vi "test_Bitfile Reload_Speciality IO Data Type Change.vi"(8 "error in (no error)":errorcluster, 11 "TestCase in":refnum<class "FPGA Addon Bitfile Reload Unit Tests.lvclass">) -> (0 "error out":errorcluster, 3 "TestCase out":refnum<class "FPGA Addon Bitfile Reload Unit Tests.lvclass">)   [LabVIEW 2020, in "FPGA Addon Bitfile Reload Unit Tests.lvclass"]
uses:
  FPGA Addon Bitfile Reload Unit Tests.lvclass
  APIs/Scripting API/TypeDefs/Output Scalar Data.ctl
  Addon/Addon Shared/Types/FPGA Addon Data Type.ctl
  APIs/Scripting API/Public/Bitfile Resources/Import Bitfile Scalars (Instances)/Import Scalars - all.vi
  <vilib>/addons/_JKI Toolkits/VI Tester/TestCase.llb/TestCase.lvclass
  APIs/Scripting API/Scripting API.lvlib
  FPGA Addon Test Class/FPGA Addon Test Class.lvclass
  Addon/Addon System Explorer/FPGA Addon System Explorer.lvlib
  Addon/Addon Shared/FPGA Addon Shared.lvlib
  C:/Program Files (x86)/National Instruments/LabVIEW 2020/vi.lib/addons/_JKI Toolkits/VI Tester/TestCase.llb/TestCase.lvclass
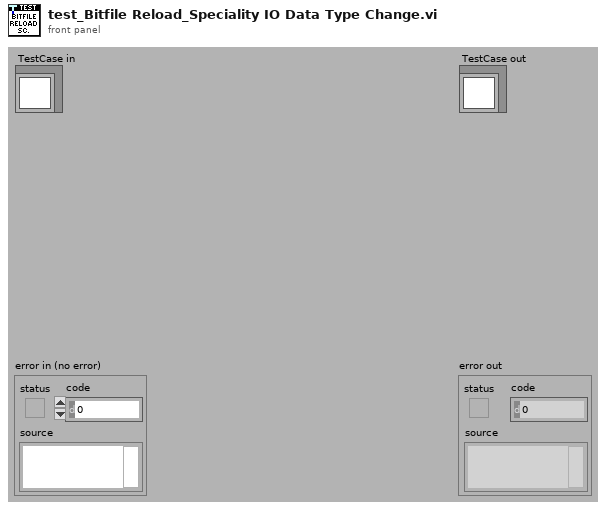
[diagram p1: front panel]
types:
  T1 = typedef "Scripting API.lvlib/Output Scalar Data.ctl" = cluster{"Bitfile Name":string, "SysDef Channel Name":string, "Imported":bool, "Data Type":T2}
  T2 = typedef "FPGA Addon Shared.lvlib/FPGA Addon Data Type.ctl" = enum8{"<Null>", "I8", "I16", "I32", "I64", "U8", "U16", "U32", "U64", "SGL", "Boolean", "Analog PWM In Settings", "Analog PWM In", "Digital PWM In Settings", "Digital PWM In", "Digital PWM Out", "Sine Out", "FXP", "FXP+/-24.5", "FXP+/-16.5", "FXP+/-32.8", "FXP+/-64.32", "FXP+/-16.7", "FXP+/-20.5", "FXP+/-27.5", "FXP+/-32.16", "FXP+16.3", "FXP+18.3", "Digital Static In", "Digital Static Out", "Digital Static In Settings", "Digital WSS Out", "Quad Encoder Settings", "Quad Encoder In", "Group"}
  T3 = typedef "Custom Device API.lvlib/Custom Device Item Ref.ctl" = u64
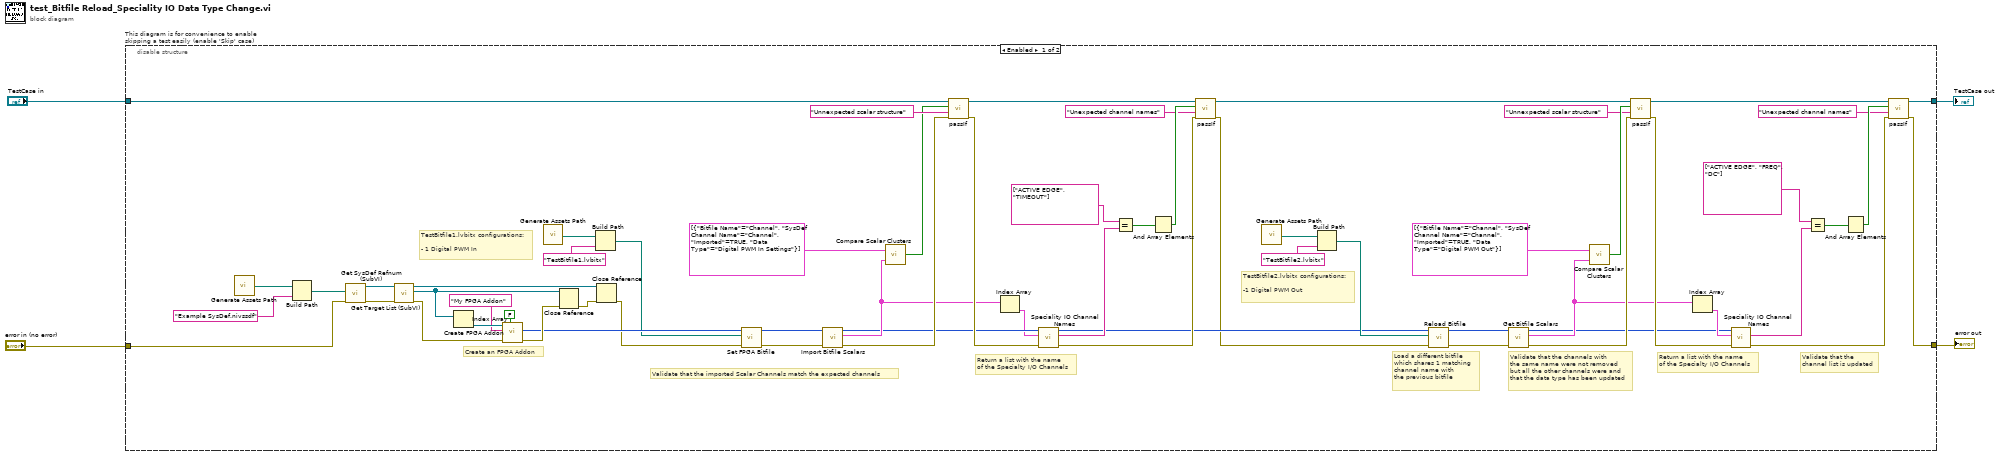
[diagram p0: block diagram]
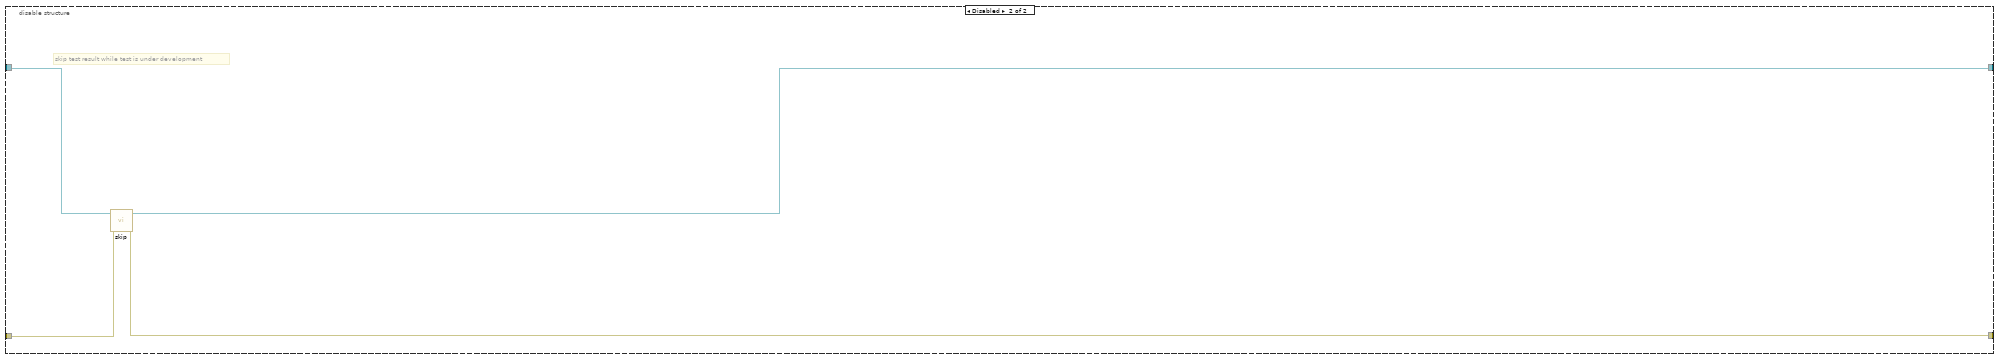
[diagram p2: hidden frame]
diagram:
  n1 = disable-structure "This diagram is for convenience to enable skipping a test easily (enable 'Skip' case)" shown="Enabled" {
    disable-tunnel: "TestCase in" -> [w35 w70]
    disable-tunnel: [w6 w68] -> w1
    disable-tunnel: [w7 w69] -> w3
    disable-tunnel: "error in (no error)" -> [w34 w67]
    frame Enabled {
      # "Validate that the\nchannel list is updated"
      # "Return a list with the name \nof the Specialty I/O Channels"
      # "Return a list with the name \nof the Specialty I/O Channels"
      # "TestBitfile2.lvbitx configurations:\n\n-1 Digital PWM Out"
      # "TestBitfile1.lvbitx configurations:\n\n- 1 Digital PWM In"
      # "Validate that the channels with \nthe same name were not removed\nbut all the other channels were and\nthat the data type has been updated"
      # "Load a different bitfile\nwhich shares 1 matching\nchannel name with \nthe previous bitfile"
      # "Validate that the imported Scalar Channels match the expected channels"
      # "Create an FPGA Addon"
      n2 = call "Generate Assets Path.vi"() -> ("Assets path"=w46:path)
      n3 = Build Path(base path=w46, name or relative path="Example SysDef.nivssdf") -> (appended path=w65:path)
      n4 = call "Get SysDef Refnum (SubVI).vi"("error in (no error)"=w34, "System Definition path"=w65) -> ("error out"=w61:errorcluster, "SysDef Refnum out"=w64:refnum<k24>)  [unwired: 8 in]
      n5 = call "Get Target List (SubVI).vi"("error in (no error)"=w61, "SysDef Refnum in"=w64) -> ("error out"=w60:errorcluster, "Target List Refnums"=w59:refnum<k24>[], "SysDef Refnum out"=w58:refnum<k24>)  [unwired: 7 in]
      n6 = Index Array(array=w59) -> (element=w63:refnum<k24>)  [unwired: 1 in]
      n7 = call "Create FPGA Addon.vi"("group scalars"=FALSE, "error in"=w60, "FPGA addon name"="My FPGA Addon", "target in"=w63) -> ("error out"=w56:errorcluster, "FPGA addon refnum"=w54:T3)  [unwired: 5 in, 1 out]
      n8 = call "Generate Assets Path.vi"() -> ("Assets path"=w45:path)
      n9 = Close Reference(reference=w59, error in (no error)=w56) -> (error out=w57:errorcluster)
      n10 = Build Path(base path=w45, name or relative path="TestBitfile1.lvbitx") -> (appended path=w51:path)
      n11 = Close Reference(reference=w58, error in (no error)=w57) -> (error out=w53:errorcluster)
      n12 = call "Set FPGA Bitfile.vi"("error in"=w53, "FPGA bitfile path"=w51, "FPGA addon refnum in"=w54) -> ("error out"=w50:errorcluster, "FPGA addon refnum out"=w49:T3)  [unwired: 7 in]
      n13 = call-poly "Import Bitfile Scalars.vi"("error in"=w50, "FPGA addon refnum in"=w49) -> ("error out"=w48:errorcluster, "imported bitfile scalars out"=w30:T1[], "FPGA addon refnum out"=w29:T3)  [unwired: 7 in]
      n14 = call "Compare Scalar Clusters.vi"("Target bitfile scalars in"=w30, "Reference bitfile scalars in"=T1[] [{"Bitfile Name"="Channel", "SysDef Channel Name"="Channel", "Imported"=TRUE, "Data Type"=enum."Digital PWM In Settings"}] ("imported bitfile scalars out")) -> ("Equal ?"=w44:bool)
      n15 = call-dynamic "passIf.vi"("error in (no error)"=w48, "message (\"\")"="Unnexpected scalar structure" ("message (\"\")"), "pass"=w44, "TestCase in"=w35) -> ("error out"=w31:errorcluster, "TestCase out"=w27:refnum<class "FPGA Addon Bitfile Reload Unit Tests.lvclass">)  [unwired: 6 in]
      n16 = Index Array(array=w30) -> (element=w28:T1)  [unwired: 1 in]
      n17 = call "Speciality IO Channel Names.vi"("error in (no error)"=w31, "channel in"=w28, "FPGA Addon ref in"=w29) -> ("error out"=w26:errorcluster, "channel names out"=w25:string[], "FPGA Addon ref out"=w20:T3)  [unwired: 6 in]
      n18 = Equal?(x=string[] ["ACTIVE EDGE", "TIMEOUT"], y=w25) -> (x = y?=w23:bool[])
      n19 = And Array Elements(Boolean array=w23) -> (logical AND=w22:bool)
      n20 = call-dynamic "passIf.vi"("error in (no error)"=w26, "message (\"\")"="Unexpected channel names" ("message (\"\")"), "pass"=w22, "TestCase in"=w27) -> ("error out"=w19:errorcluster, "TestCase out"=w18:refnum<class "FPGA Addon Bitfile Reload Unit Tests.lvclass">)  [unwired: 6 in]
      n21 = call "Generate Assets Path.vi"() -> ("Assets path"=w42:path)
      n22 = Build Path(base path=w42, name or relative path="TestBitfile2.lvbitx") -> (appended path=w41:path)
      n23 = call "Reload Bitfile.vi"("error in (no error)"=w19, "NewVal"=w41, "Item Ref in"=w20) -> ("error out"=w40:errorcluster, "Section Ref out"=w39:T3)  [unwired: 7 in]
      n24 = call "Get Bitfile Scalars.vi"("error in"=w40, "FPGA addon refnum in"=w39) -> ("error out"=w38:errorcluster, "bitfile scalars out"=w8:T1[], "FPGA addon refnum out"=w5:T3)  [unwired: 7 in]
      n25 = call "Compare Scalar Clusters.vi"("Target bitfile scalars in"=w8, "Reference bitfile scalars in"=T1[] [{"Bitfile Name"="Channel", "SysDef Channel Name"="Channel", "Imported"=TRUE, "Data Type"=enum."Digital PWM Out"}] ("bitfile scalars out")) -> ("Equal ?"=w37:bool)
      n26 = call-dynamic "passIf.vi"("error in (no error)"=w38, "message (\"\")"="Unnexpected scalar structure" ("message (\"\")"), "pass"=w37, "TestCase in"=w18) -> ("error out"=w9:errorcluster, "TestCase out"=w10:refnum<class "FPGA Addon Bitfile Reload Unit Tests.lvclass">)  [unwired: 6 in]
      n27 = Index Array(array=w8) -> (element=w17:T1)  [unwired: 1 in]
      n28 = call "Speciality IO Channel Names.vi"("error in (no error)"=w9, "channel in"=w17, "FPGA Addon ref in"=w5) -> ("error out"=w16:errorcluster, "channel names out"=w15:string[])  [unwired: 6 in, 1 out]
      n29 = Equal?(x=string[] ["ACTIVE EDGE", "FREQ", "DC"], y=w15) -> (x = y?=w13:bool[])
      n30 = And Array Elements(Boolean array=w13) -> (logical AND=w12:bool)
      n31 = call-dynamic "passIf.vi"("error in (no error)"=w16, "message (\"\")"="Unexpected channel names" ("message (\"\")"), "pass"=w12, "TestCase in"=w10) -> ("error out"=w7:errorcluster, "TestCase out"=w6:refnum<class "FPGA Addon Bitfile Reload Unit Tests.lvclass">)  [unwired: 6 in]
    }
    frame Disabled {
      # "skip test result while test is under development"
      n32 = call <vilib>:"skip.vi"("error in (no error)"=w67, "TestCase in"=w70) -> ("error out"=w69:errorcluster, "TestCase out"=w68:refnum<class "FPGA Addon Bitfile Reload Unit Tests.lvclass">)  [unwired: 8 in]
    }
  }
  "error out" <- w3
  "TestCase out" <- w1
